vi "Ex. 4. Build Your First Application.vi"() -> ()   [LabVIEW 2024]
uses:
  <vilib>/measure/NI_MABase.lvlib
panel:
  out "Processed Data":waveform(dbl)(graph)
  in  "Stop":bool
  in  "Frequency":dbl(knob) scale=0.0..50.0
  out "Original Data":waveform(dbl)(graph)
  # "Signal Generation Demo"
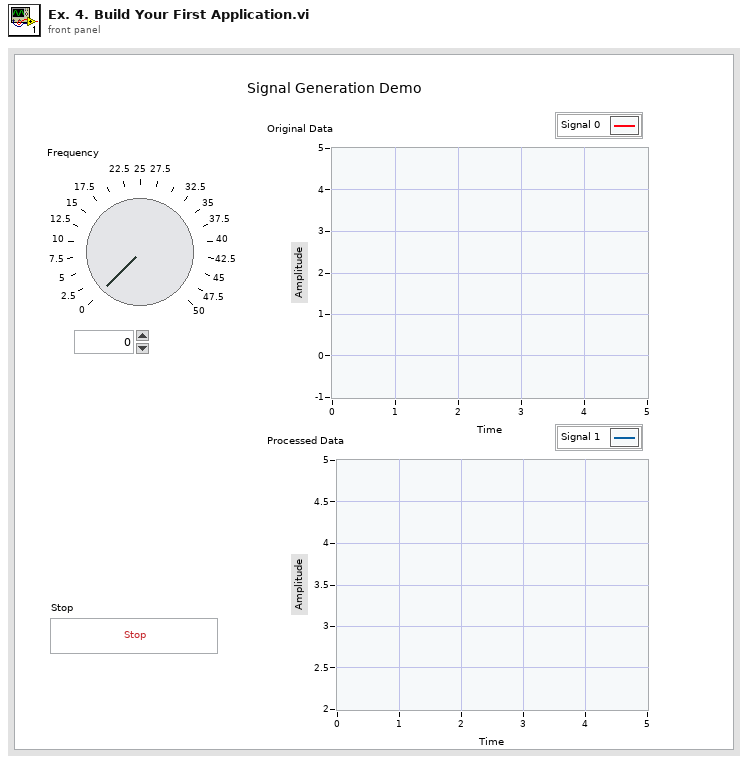
[diagram p1: front panel]
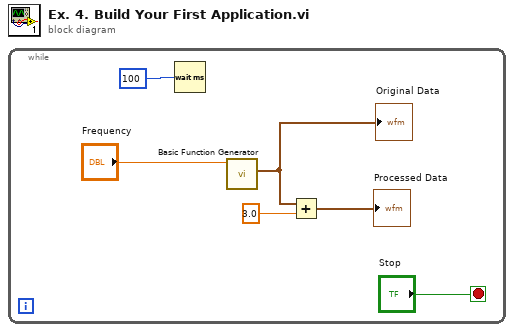
[diagram p0: block diagram]
diagram:
  n1 = while {
    stop <- "Stop" stop-if-true
    n2 = Wait (ms)(milliseconds to wait=u32 100) -> ()  [unwired: 1 out]
    n3 = call <vilib>:"Basic Function Generator.vi"("frequency"="Frequency") -> ("signal out"=w3:waveform(dbl))  [unwired: 8 in, 2 out]
    "Original Data" <- w3
    n4 = Add(x=w3, y=3.0) -> (x+y=→"Processed Data":waveform(dbl))
  }
